vi "fgv_Sys and HW Config.vi"(5 "Standalone viewer initialisation?":bool, 6 "backup file path":path, 7 "Function":T21, 8 "error in (no error)":errorcluster, 10 "System Config":T1={"Laser wavelength (nm)"=920.0, "DAQ FPGA System"={"Clock Freq (MHz) "=200.0, "Samples Wait after Trigger"=5080, "AOD fill"=4900, "StartupDelay"=0, "Slip Cycle (clock cycles)"=600000, "Add Cycle"=TRUE}, "Control system"={"AOD 1 Amplitude"=0, "AOD 2 Amplitude"=0, "AOD 3 Amplitude"=0, "AOD 4 Amplitude"=0, "AOD 5 Amplitude"=0, "AOD 6 Amplitude"=0, "T0 (ns)"=0.0, "Ta (ns)"=0.0, "Data Time Interval (ns)"=0.0, "Ctrl FPGA Clock (MHz)"=240.0}} {"Control system"."Ctrl FPGA Clock (MHz)" min=80.0 max=500.0 step=1.0; "Control system"."Data Time Interval (ns)" min=0.0 max=2048.0 step=1.0; "Control system"."Ta (ns)" min=0.0 max=2048.0 step=1.0; "Control system"."T0 (ns)" min=0.0 max=2048.0 step=1.0; "Control system"."AOD 6 Amplitude" min=0 max=2048 step=1; "Control system"."AOD 5 Amplitude" min=0 max=2048 step=1; "Control system"."AOD 4 Amplitude" min=0 max=2048 step=1; "Control system"."AOD 3 Amplitude" min=0 max=2048 step=1; "Control system"."AOD 2 Amplitude" min=0 max=2048 step=1; "Control system"."AOD 1 Amplitude" min=0 max=2048 step=1; "Laser wavelength (nm)" min=800.0 max=1080.0 step=1.0}, 11 "Hardware Configuration":T4={"Dev. PC"=FALSE, "Swap XY on stage"=FALSE, "No of AOD"=0, "MC Supported"=FALSE, "Axial MC"=FALSE, "Computer MAC address"="", "Externalise Triggers"=FALSE, "Trigger HW config"={"Available Device List"=0, "Device Address"=""}, "DAQmx Chan"={"Pockels AO"="", "Hard shutter AO"="", "PMT AOs"="", "Galvo AOs"="", "Power meter AI"=""}, "XYZ Stage Control Config"=enum."None", "XY stage available"=FALSE, "XY Comms Config Cluster"={"Name"="COM7", "Device Address"="", "Port "=0, "Baudrate"=0, "Comms Type"=enum."GPIB-IEEE488"}, "Y stage available"=FALSE, "Y Comms Config Cluster"={"Name"="", "Device Address"="", "Port "=0, "Baudrate"=0, "Comms Type"=enum."GPIB-IEEE488"}, "Z stage available"=FALSE, "Z Comms Config Cluster "={"Name"="", "Device Address"="", "Port "=0, "Baudrate"=0, "Comms Type"=enum."GPIB-IEEE488"}, "Encoder available"=FALSE, "Encoder"={"IP address"="224.0.1.103", "Port"=7000, "Wheel radius (cm)"=16.0, "Encoder Trigger"=""}, "VidRec available"=FALSE, "Cam VidRec"={"DO flag-Video record"="", "DO flag-Trial start"=""}, "Laser Power Control HW config"={"Laser Power Control"="", "Laser Power Modulation Control"=enum."NI"}, "Laser 1 available"=FALSE, "Laser 1 config cluster"={"COM port"="COM7", "Baud Rate"=0, "Type"=""}, "Prechirper 1 available"=FALSE, "Prechirper 1 config cluster"={"Type"="", "Baud Rate"=0, "COM port"="COM7"}, "Control system.FPGA available?"=FALSE, "Control Sys. HW config"={"Control system.FPGA Type"=enum."Virtex 5", "Control system.Network adapter name"="", "Control system.MAC address"="", "Control system.Ethernet Port"=0, "Control system.Ethernet Port Opened"=FALSE}, "DAQ FPGA HW Config"={"FGPA Ref"=refnum, "Target"="RIO0", "input card type"=enum."AC Card"}, "PMT Control Voltage Limits"={"Lower Limit"=0.0, "Upper Limit"=0.0}} {"Encoder"."Wheel radius (cm)" format="%#_13g"}) -> (0 "error out":errorcluster, 2 "System Config OUT":T1={"Laser wavelength (nm)"=920.0, "DAQ FPGA System"={"Clock Freq (MHz) "=200.0, "Samples Wait after Trigger"=5080, "AOD fill"=4900, "StartupDelay"=0, "Slip Cycle (clock cycles)"=600000, "Add Cycle"=TRUE}, "Control system"={"AOD 1 Amplitude"=0, "AOD 2 Amplitude"=0, "AOD 3 Amplitude"=0, "AOD 4 Amplitude"=0, "AOD 5 Amplitude"=0, "AOD 6 Amplitude"=0, "T0 (ns)"=0.0, "Ta (ns)"=0.0, "Data Time Interval (ns)"=0.0, "Ctrl FPGA Clock (MHz)"=240.0}} {"Control system"."Ctrl FPGA Clock (MHz)" min=80.0 max=500.0 step=1.0; "Control system"."Data Time Interval (ns)" min=0.0 max=2048.0 step=1.0; "Control system"."Ta (ns)" min=0.0 max=2048.0 step=1.0; "Control system"."T0 (ns)" min=0.0 max=2048.0 step=1.0; "Control system"."AOD 6 Amplitude" min=0 max=2048 step=1; "Control system"."AOD 5 Amplitude" min=0 max=2048 step=1; "Control system"."AOD 4 Amplitude" min=0 max=2048 step=1; "Control system"."AOD 3 Amplitude" min=0 max=2048 step=1; "Control system"."AOD 2 Amplitude" min=0 max=2048 step=1; "Control system"."AOD 1 Amplitude" min=0 max=2048 step=1; "Laser wavelength (nm)" min=800.0 max=1080.0 step=1.0}, 3 "Hardware Configuration OUT":T4={"Dev. PC"=FALSE, "Swap XY on stage"=FALSE, "No of AOD"=0, "MC Supported"=FALSE, "Axial MC"=FALSE, "Computer MAC address"="", "Externalise Triggers"=FALSE, "Trigger HW config"={"Available Device List"=0, "Device Address"=""}, "DAQmx Chan"={"Pockels AO"="", "Hard shutter AO"="", "PMT AOs"="", "Galvo AOs"="", "Power meter AI"=""}, "XYZ Stage Control Config"=enum."None", "XY stage available"=FALSE, "XY Comms Config Cluster"={"Name"="COM7", "Device Address"="", "Port "=0, "Baudrate"=0, "Comms Type"=enum."GPIB-IEEE488"}, "Y stage available"=FALSE, "Y Comms Config Cluster"={"Name"="", "Device Address"="", "Port "=0, "Baudrate"=0, "Comms Type"=enum."GPIB-IEEE488"}, "Z stage available"=FALSE, "Z Comms Config Cluster "={"Name"="", "Device Address"="", "Port "=0, "Baudrate"=0, "Comms Type"=enum."GPIB-IEEE488"}, "Encoder available"=FALSE, "Encoder"={"IP address"="224.0.1.103", "Port"=7000, "Wheel radius (cm)"=16.0, "Encoder Trigger"=""}, "VidRec available"=FALSE, "Cam VidRec"={"DO flag-Video record"="", "DO flag-Trial start"=""}, "Laser Power Control HW config"={"Laser Power Control"="", "Laser Power Modulation Control"=enum."NI"}, "Laser 1 available"=FALSE, "Laser 1 config cluster"={"COM port"="COM7", "Baud Rate"=0, "Type"=""}, "Prechirper 1 available"=FALSE, "Prechirper 1 config cluster"={"Type"="", "Baud Rate"=0, "COM port"="COM7"}, "Control system.FPGA available?"=FALSE, "Control Sys. HW config"={"Control system.FPGA Type"=enum."Virtex 5", "Control system.Network adapter name"="", "Control system.MAC address"="", "Control system.Ethernet Port"=0, "Control system.Ethernet Port Opened"=FALSE}, "DAQ FPGA HW Config"={"FGPA Ref"=refnum, "Target"="RIO0", "input card type"=enum."AC Card"}, "PMT Control Voltage Limits"={"Lower Limit"=0.0, "Upper Limit"=0.0}} {"Encoder"."Wheel radius (cm)" format="%#_13g"})   [LabVIEW 2020]
uses:
  Typedefs/Save-Load enum.ctl
  General Globals.vi
  <vilib>/userDefined/High Color/nirio_resource_hc.ctl
  Typedefs/DAQmx physical channels cluster.ctl
  Typedefs/HW config states enum.ctl
  RIG-SPECIFIC FILES/FPGA Refs/FPGA Ref.ctl
  Typedefs/FPGA input type AC-DC.ctl
  Typedefs/Encoder config cluster.ctl
  Typedefs/Cam VidRec HW config setup cluster.ctl
  Typedefs/DAQ FPGA system config.ctl
  Typedefs/CTRL system config.ctl
  Typedefs/System Configuration.ctl
  Typedefs/Control Sys HW config cluster.ctl
  Typedefs/Triggers HW config.ctl
  Typedefs/Laser 1 config cluster.ctl
  Typedefs/PreChirper 1 config cluster.ctl
  Typedefs/Laser Power Control HW config.ctl
  Typedefs/Hardware Configuration settings.ctl
  Typedefs/DAQ FPGA HW config cluster.ctl
  Typedefs/PMT Control Voltage limits.ctl
  Peripherals Control/XYZ Stage/Control/typedefs/XYZControlConfig.ctl
  Typedefs/Comms Type.ctl
  Typedefs/Peripherals comms config cluster.ctl
panel:
  # "FUNCTIONAL GLOBAL"
  # "<--- The \"PMT AOs\" DAQmx string will always contain\n                       2 channels is this format: PXI1Slot4/ao2:3"
  # "(make , model etc)"
  # "(COM Port / IP Address / service address etc.)"
  # "(Port for ethernet / channel for BT)"
  # "(make , model etc)"
  # "(COM Port / IP Address / service address etc.)"
  # "(Port for ethernet / channel for BT)"
  # "(make , model etc)"
  # "(COM Port / IP Address / service address etc.)"
  # "(Port for ethernet / channel for BT)"
  # "(make , model etc)"
  # "(COM Port / IP Address / service address etc.)"
  # "(Port for ethernet / channel for BT)"
  # "(make , model etc)"
  # "(COM Port / IP Address / service address etc.)"
  # "(Port for ethernet / channel for BT)"
  # "(make , model etc)"
  # "(COM Port / IP Address / service address etc.)"
  # "(Port for ethernet / channel for BT)"
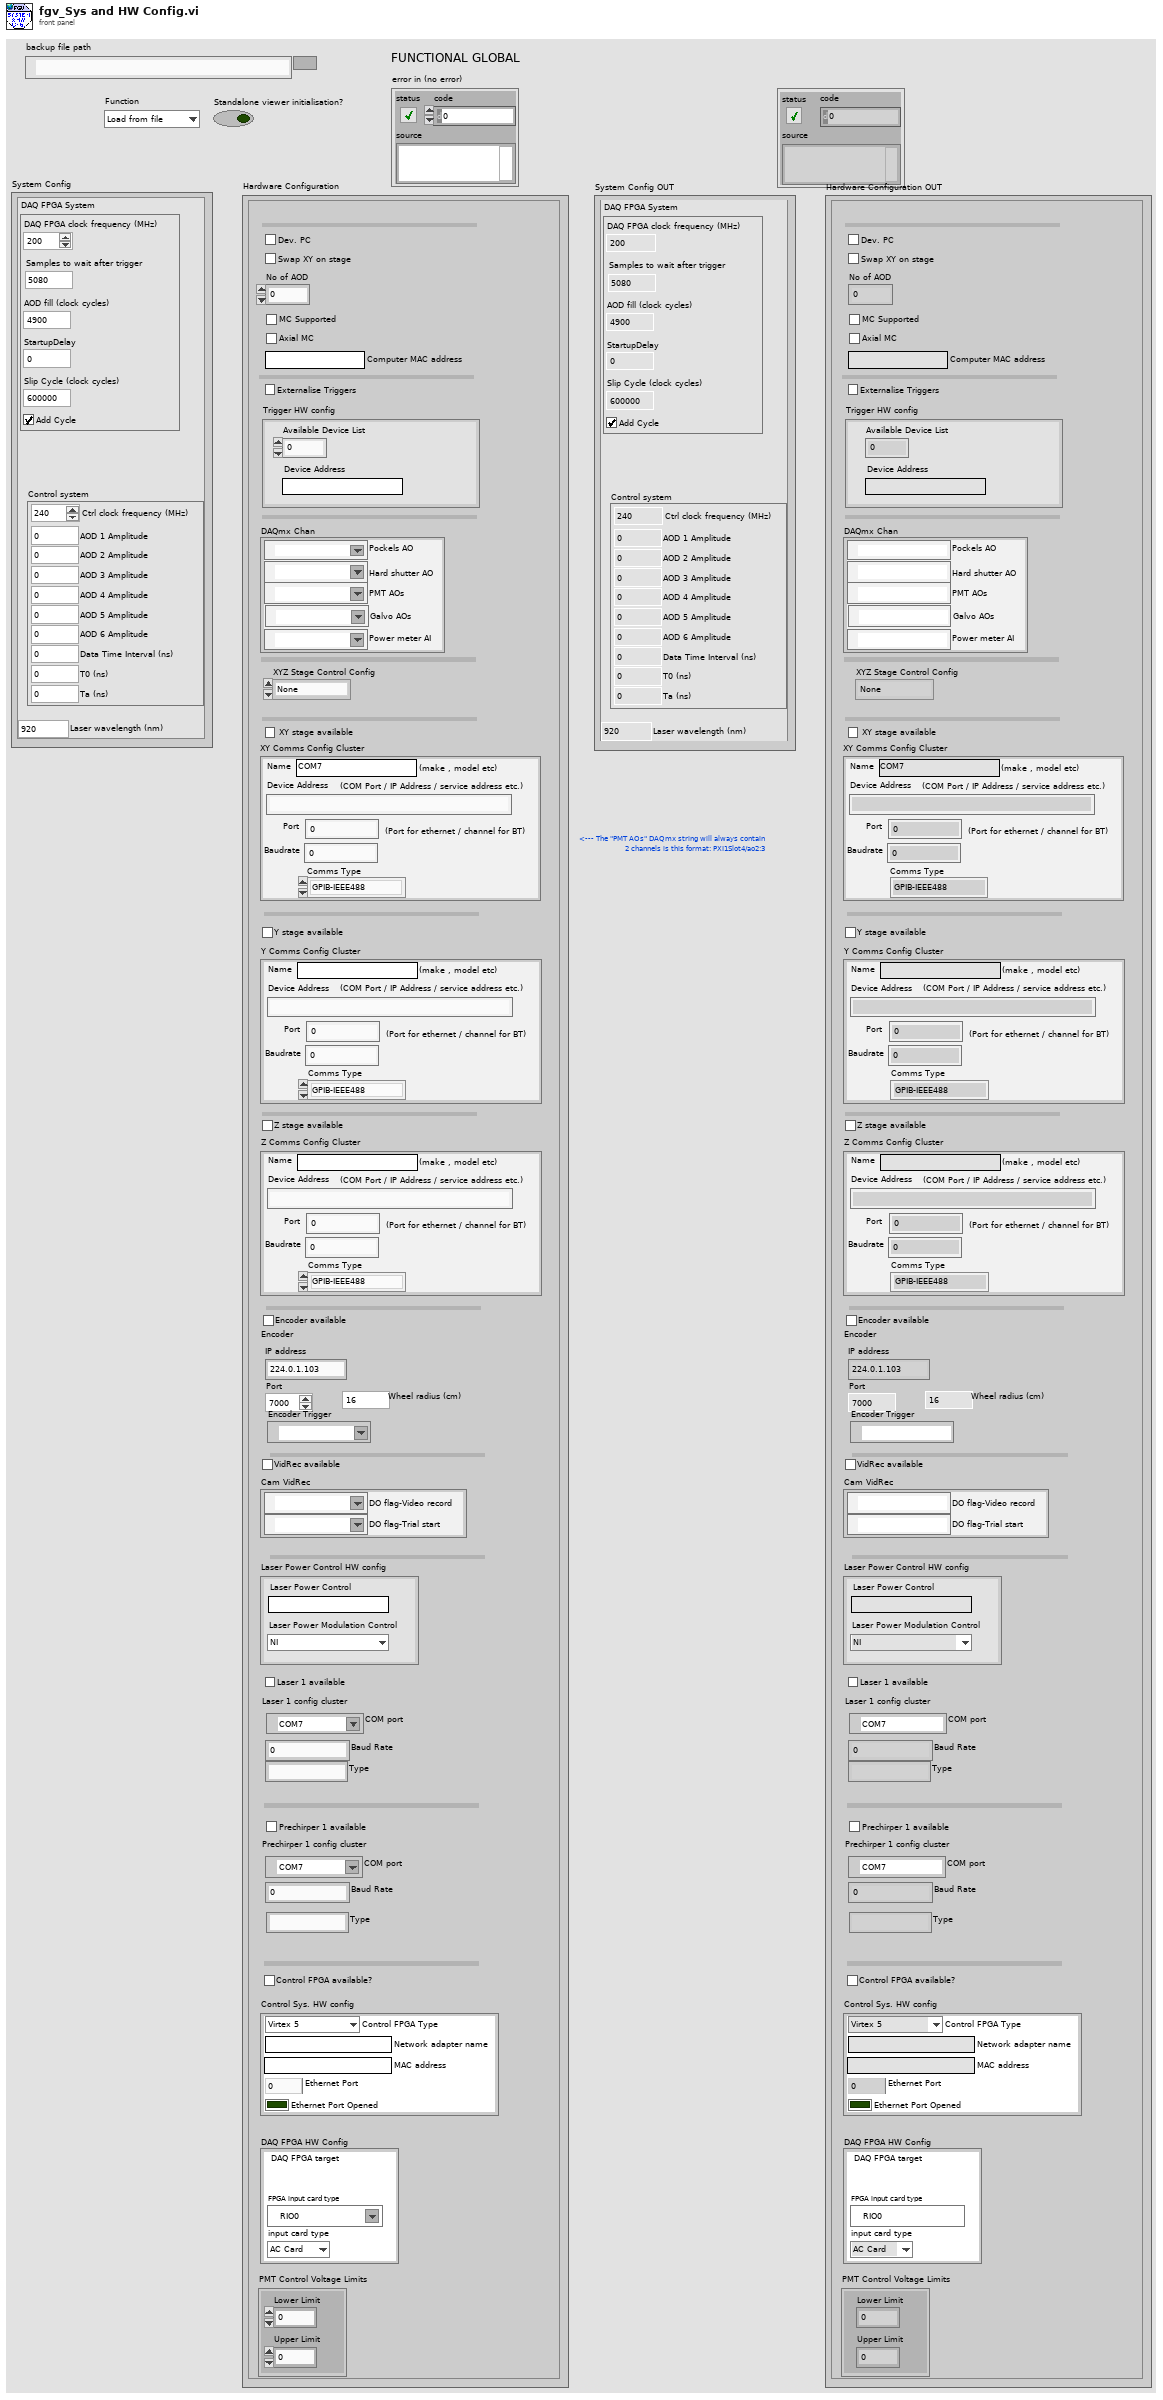
[diagram p1: front panel]
types:
  T1 = typedef "System Configuration.ctl" = cluster{"Laser wavelength (nm)":dbl, "DAQ FPGA System":T2, "Control system":T3}
  T2 = typedef "DAQ FPGA system config.ctl" = cluster{"Clock Freq (MHz) ":dbl, "Samples Wait after Trigger":u16, "AOD fill":u16, "StartupDelay":i32, "Slip Cycle (clock cycles)":u32, "Add Cycle":bool}
  T3 = typedef "CTRL system config.ctl" = cluster{"AOD 1 Amplitude":i16, "AOD 2 Amplitude":i16, "AOD 3 Amplitude":i16, "AOD 4 Amplitude":i16, "AOD 5 Amplitude":i16, "AOD 6 Amplitude":i16, "T0 (ns)":dbl, "Ta (ns)":dbl, "Data Time Interval (ns)":dbl, "Ctrl FPGA Clock (MHz)":dbl}
  T4 = typedef "Hardware Configuration settings.ctl" = cluster{"Dev. PC":bool, "Swap XY on stage":bool, "No of AOD":u8, "MC Supported":bool, "Axial MC":bool, "Computer MAC address":string, "Externalise Triggers":bool, "Trigger HW config":T5, "DAQmx Chan":T6, "XYZ Stage Control Config":T7, "XY stage available":bool, "XY Comms Config Cluster":T8, "Y stage available":bool, "Y Comms Config Cluster":T8, "Z stage available":bool, "Z Comms Config Cluster ":T8, "Encoder available":bool, "Encoder":T10, "VidRec available":bool, "Cam VidRec":T11, "Laser Power Control HW config":T12, "Laser 1 available":bool, "Laser 1 config cluster":T13, "Prechirper 1 available":bool, "Prechirper 1 config cluster":T14, "Control system.FPGA available?":bool, "Control Sys. HW config":T15, "DAQ FPGA HW Config":T16, "PMT Control Voltage Limits":T20}
  T5 = typedef "Triggers HW config.ctl" = cluster{"Available Device List":i32, "Device Address":string}
  T6 = typedef "DAQmx physical channels cluster.ctl" = cluster{"Pockels AO":tag, "Hard shutter AO":tag, "PMT AOs":tag, "Galvo AOs":tag, "Power meter AI":tag}
  T7 = typedef "XYZControlConfig.ctl" = enum16{"None", "XYZ", "XY-Z", "X-Y-Z", "Z"}
  T8 = typedef "Peripherals comms config cluster.ctl" = cluster{"Name":string, "Device Address":string, "Port ":u16, "Baudrate":i32, "Comms Type":T9}
  T9 = typedef "Comms Type.ctl" = enum16{"GPIB-IEEE488", "Serial-RS232", "Serial-RS485", "Serial-RS422", "Serial-USB", "Ethernet-TCP/IP", "Ethernet-UDP"}
  T10 = typedef "Encoder config cluster.ctl" = cluster{"IP address":string, "Port":u16, "Wheel radius (cm)":dbl, "Encoder Trigger":tag}
  T11 = typedef "Cam VidRec HW config setup cluster.ctl" = cluster{"DO flag-Video record":tag, "DO flag-Trial start":tag}
  T12 = typedef "Laser Power Control HW config.ctl" = cluster{"Laser Power Control":string, "Laser Power Modulation Control":enum16{"NI", "FPGA"}}
  T13 = typedef "Laser 1 config cluster.ctl" = cluster{"COM port":refnum<visa-resource-name>, "Baud Rate":i32, "Type":string}
  T14 = typedef "PreChirper 1 config cluster.ctl" = cluster{"Type":string, "Baud Rate":i32, "COM port":refnum<visa-resource-name>}
  T15 = typedef "Control Sys HW config cluster.ctl" = cluster{"Control system.FPGA Type":enum16{"Virtex 5", "Virtex 7"}, "Control system.Network adapter name":string, "Control system.MAC address":string, "Control system.Ethernet Port":u32, "Control system.Ethernet Port Opened":bool}
  T16 = typedef "DAQ FPGA HW config cluster.ctl" = cluster{"FGPA Ref":T17, "Target":T18, "input card type":T19}
  T17 = typedef "FPGA Ref.ctl" = refnum<k20>
  T18 = typedef "nirio_resource_hc.ctl" = tag
  T19 = typedef "FPGA input type AC-DC.ctl" = enum16{"AC Card", "DC Card"}
  T20 = typedef "PMT Control Voltage limits.ctl" = cluster{"Lower Limit":dbl, "Upper Limit":dbl}
  T21 = typedef "HW config states enum.ctl" = enum16{"Load from file", "Save to file", "Save backup", "Write all", "Read all", "Write XY stage settings", "Write DAQ FPGA settings", "Write Control FPGA settings", "Write Phys Channels", "Write System Config", "Write HW Config", "Save System Config", "Save HW Config", "Clear", "Compare from file"}
  T22 = typedef "Save-Load enum.ctl" = enum16{"Save to file", "Load from file", "Compare from file", "Save Backup"}
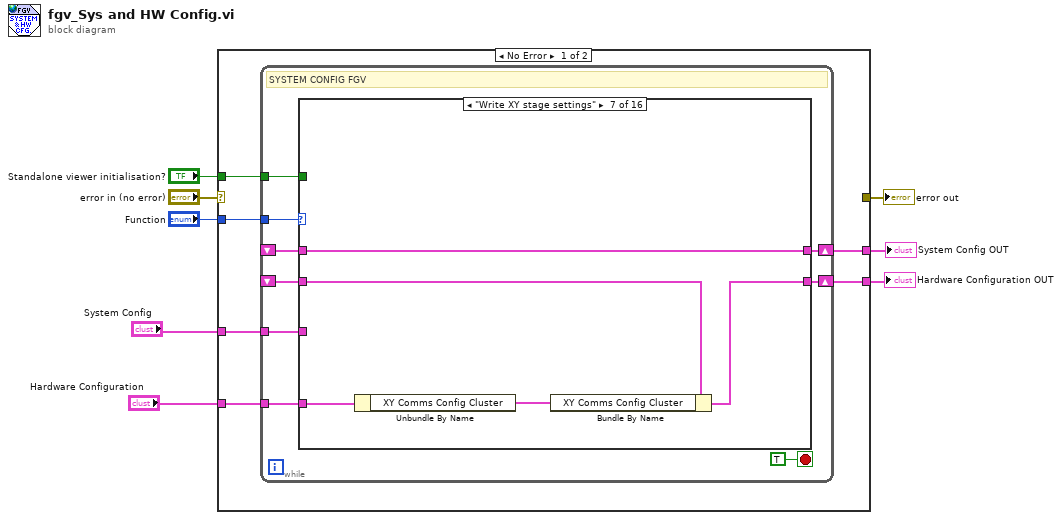
[diagram p0: block diagram]
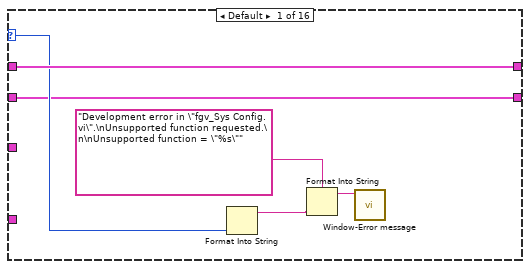
[diagram p2: hidden frame]
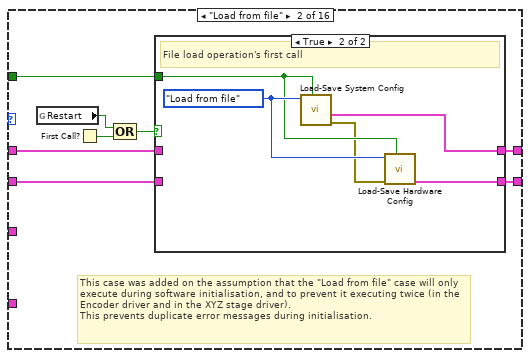
[diagram p3: hidden frame]
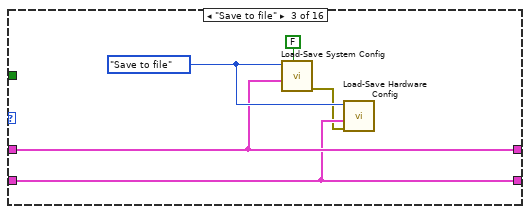
[diagram p5: hidden frame]
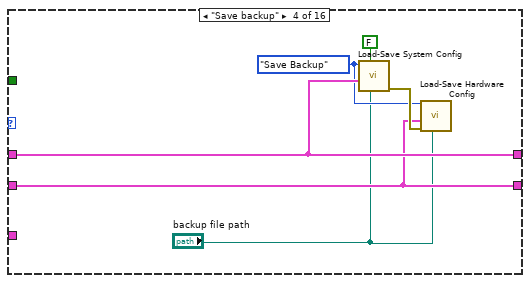
[diagram p6: hidden frame]
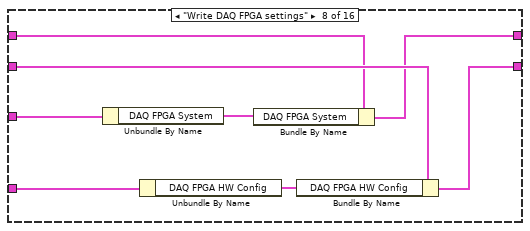
[diagram p9: hidden frame]
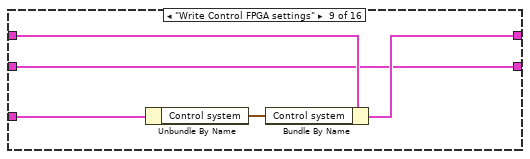
[diagram p10: hidden frame]
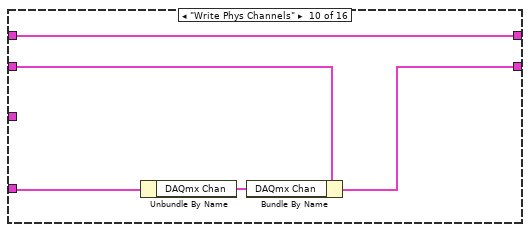
[diagram p11: hidden frame]
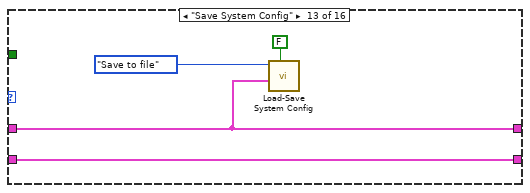
[diagram p14: hidden frame]
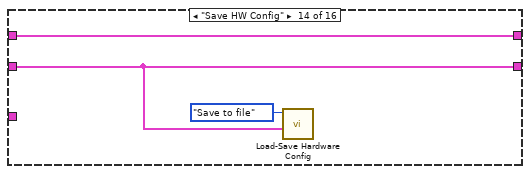
[diagram p15: hidden frame]
diagram:
  n1 = case shown="No Error" "error in (no error)" {
    selector: "error in (no error)" -> [_ w96]
    tunnel: [_ w96] -> w7
    tunnel: "Function" -> [w14 _]
    tunnel: "System Config" -> [w13 _]
    tunnel: [w12 _] -> w1
    tunnel: "Standalone viewer initialisation?" -> [w11 _]
    tunnel: "Hardware Configuration" -> [w10 _]
    tunnel: [w9 _] -> w2
    frame No Error {
      n2 = while {
        tunnel: w14 -> [w23]
        shift-right: [w21] -> w12
        shift-left: _ -> [w19]
        tunnel: w13 -> [w20]
        tunnel: w11 -> [w18]
        tunnel: w10 -> [w17]
        shift-right: [w16] -> w9
        shift-left: _ -> [w15]
        stop <- TRUE stop-if-true
        # "SYSTEM CONFIG FGV"
        n3 = case shown="\"Write XY stage settings\"" w23 {
          selector: w23 -> [w25 _ _ _ _ _ _ _ _ _ _ _ _ _ _ _]
          tunnel: [w26 w32 w47 w53 w57 w59 w60 w66 w74 w81 w83 w86 w87 w93 w95 _] -> w21
          tunnel: w20 -> [_ _ _ _ w57 _ _ w68 w77 _ w83 _ _ _ _ _]
          tunnel: w19 -> [w26 w37 w47 w53 _ w59 w60 w67 w76 w81 _ w86 w87 w93 w95 _]
          tunnel: w18 -> [_ w33 _ _ _ _ _ _ _ _ _ _ _ _ _ _]
          tunnel: w17 -> [_ _ _ _ w56 _ w63 w71 _ w80 _ w85 _ _ _ _]
          tunnel: [w24 w31 w46 w52 w56 w58 w61 w69 w73 w78 w84 w85 w90 w91 w94 _] -> w16
          tunnel: w15 -> [w24 w30 w46 w52 _ w58 w62 w70 w73 w79 w84 _ w90 w91 w94 _]
          frame Default {
            n4 = Format Into String(w25) -> (resulting string=w28:string)  [unwired: 3 in, 1 out]
            n5 = Format Into String(format string="Development error in \"fgv_Sys Config.vi\".\nUnsupported function requested.\n\nUnsupported function = \"%s\"" ("Message"), w28) -> (resulting string=w27:string)  [unwired: 2 in, 1 out]
            n6 = call "Window-Error message.vi"("Message"=w27) -> ()  [unwired: 10 in, 1 out]
          }
          frame "Load from file" {
            # "This case was added on the assumption that the \"Load from file\" case will only execute during software initialisation, and to prevent it executing twice (in the Encoder driver and in the XYZ stage driver).\nThis prevents duplicate error messages during initialisation."
            n7 = global read "General Globals.vi" "Restart"() -> (w34:bool)
            n8 = First Call?() -> (First Call?: T/F=w36:bool)
            n9 = Compound Arithmetic op=OR(w34, w36) -> (w35:bool)
            n10 = case shown="True" w35 {
              tunnel: w37 -> [w39 _]
              tunnel: w33 -> [_ w41]
              tunnel: [w39 w44] -> w32
              tunnel: [w38 w42] -> w31
              tunnel: w30 -> [w38 _]
              frame False {
                # "Already loaded"
              }
              frame True {
                w43 = Save-Load_enum."Load from file" ("Function")
                # "File load operation's first call"
                n11 = call "Load-Save System Config.vi"("Standalone viewer?"=w41, "Function"=w43) -> ("error out"=w40:errorcluster, "System Config O/P"=w44:T1)  [unwired: 8 in]
                n12 = call "Load-Save Hardware Config.vi"("Standalone ?"=w41, "error in"=w40, "Function"=w43) -> ("Hardware Configuration O/P"=w42:T4)  [unwired: 7 in, 1 out]
              }
            }
          }
          frame "Save to file" {
            w48 = Save-Load_enum."Save to file" ("Function")
            n13 = call "Load-Save System Config.vi"("Standalone viewer?"=FALSE, "System Config I/P"=w47, "Function"=w48) -> ("error out"=w45:errorcluster)  [unwired: 7 in, 1 out]
            n14 = call "Load-Save Hardware Config.vi"("error in"=w45, "Hardware Configuration I/P"=w46, "Function"=w48) -> ()  [unwired: 7 in, 2 out]
          }
          frame "Save backup" {
            w51 = Save-Load_enum."Save Backup" ("Function")
            n15 = call "Load-Save System Config.vi"("backup file path"="backup file path", "Standalone viewer?"=FALSE, "System Config I/P"=w53, "Function"=w51) -> ("error out"=w54:errorcluster)  [unwired: 6 in, 1 out]
            n16 = call "Load-Save Hardware Config.vi"("Backup file path"="backup file path", "error in"=w54, "Hardware Configuration I/P"=w52, "Function"=w51) -> ()  [unwired: 6 in, 2 out]
          }
          frame "Write all" {
          }
          frame "Read all" {
          }
          frame "Write XY stage settings" {
            n17 = Unbundle By Name(w63) -> ("XY Comms Config Cluster"=w64:T8)
            n18 = Bundle By Name(cluster=w62, "XY Comms Config Cluster"=w64) -> (w61:T4)
          }
          frame "Write DAQ FPGA settings" {
            n19 = Unbundle By Name(w68) -> ("DAQ FPGA System"=w65:T2)
            n20 = Unbundle By Name(w71) -> ("DAQ FPGA HW Config"=w72:T16)
            n21 = Bundle By Name(cluster=w67, "DAQ FPGA System"=w65) -> (w66:T1)
            n22 = Bundle By Name(cluster=w70, "DAQ FPGA HW Config"=w72) -> (w69:T4)
          }
          frame "Write Control FPGA settings" {
            n23 = Unbundle By Name(w77) -> ("Control system"=w75:T3)
            n24 = Bundle By Name(cluster=w76, "Control system"=w75) -> (w74:T1)
          }
          frame "Write Phys Channels" {
            n25 = Unbundle By Name(w80) -> ("DAQmx Chan"=w82:T6)
            n26 = Bundle By Name(cluster=w79, "DAQmx Chan"=w82) -> (w78:T4)
          }
          frame "Write System Config" {
          }
          frame "Write HW Config" {
          }
          frame "Save System Config" {
            n27 = call "Load-Save System Config.vi"("Standalone viewer?"=FALSE, "System Config I/P"=w87, "Function"=Save-Load_enum."Save to file") -> ()  [unwired: 7 in, 2 out]
          }
          frame "Save HW Config" {
            n28 = call "Load-Save Hardware Config.vi"("Hardware Configuration I/P"=w91, "Function"=Save-Load_enum."Save to file") -> ()  [unwired: 8 in, 2 out]
          }
          frame "Compare from file" {
          }
          frame "Clear" {
          }
        }
      }
    }
    frame Error {
    }
  }
  "error out" <- w7
  "Hardware Configuration OUT" <- w2
  "System Config OUT" <- w1
